vi "Controller Build FA Blocks and Send to Fast Archiver Data Loop.vi"(5 "Number of Blocks":u32, 7 "FA Data (Zeroed)":sgl[][](array[numeric]), 8 "Timestamp":u64, 9 "FC Marker":u32, 10 "FA Data (BPM Readings / PS Readings / PS Setpoints)":dbl[](array[numeric]), 11 "Queue in":refnum<queue>) -> ()   [LabVIEW 2011, in "Controller VIs.lvlib"]
uses:
  Controller VIs.lvlib
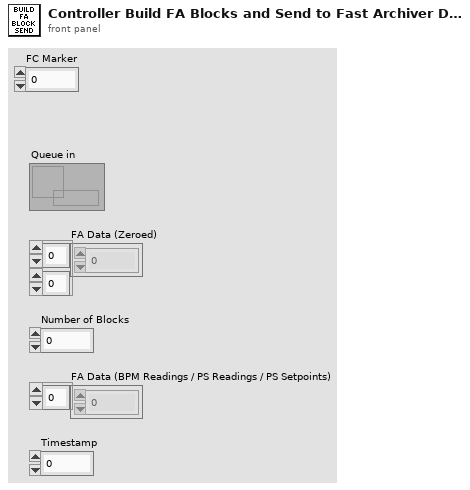
[diagram p1: front panel]
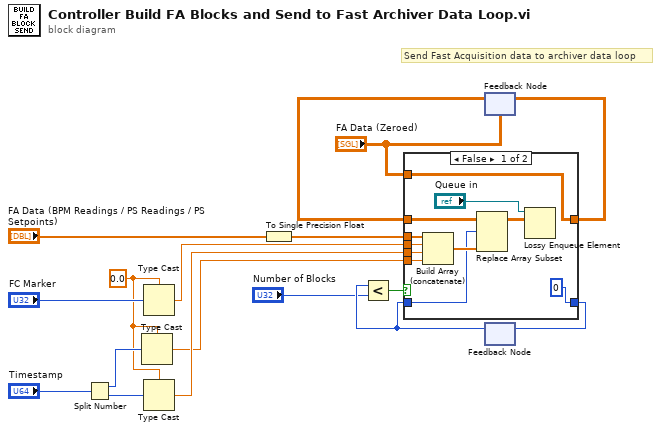
[diagram p0: block diagram]
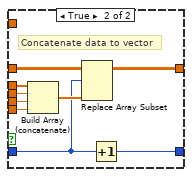
[diagram p2: hidden frame]
diagram:
  w2 = sgl 0.0 ("single precision float")
  # "Send Fast Acquisition data to archiver data loop"
  n1 = Split Number(x="Timestamp") -> (hi(x)=w15:u32, lo(x)=w14:u32)
  n2 = Type Cast(type=w2, x=w15) -> (*(type *) &x=w16:sgl)
  n3 = Type Cast(type=w2, x="FC Marker") -> (*(type *) &x=w1:sgl)
  n4 = Type Cast(type=w2, x=w14) -> (*(type *) &x=w17:sgl)
  n5 = To Single Precision Float(number="FA Data (BPM Readings / PS Readings / PS Setpoints)") -> (single precision float=w13:sgl[])
  n6 = feedback #1("FA Data (Zeroed)") -> (w7:sgl[][])
  n7 = feedback #2() -> (w11:i32)  [unwired: 1 in]
  n8 = Less?(x=w11, y="Number of Blocks") -> (x < y?=w9:bool)
  n9 = case shown="False" w9 {
    tunnel: [0 ("x+1") w35] -> w8
    tunnel: [w21 w34] -> w6
    tunnel: w7 -> [w28 w37]
    tunnel: w11 -> [w25 w33]
    tunnel: w17 -> [w19 w30]
    tunnel: w13 -> [w23 w32]
    tunnel: w16 -> [w20 w31]
    tunnel: "FA Data (Zeroed)" -> [w21 _]
    tunnel: w1 -> [w18 w29]
    frame False {
      n10 = Build Array (concatenate)(w23, w18, w19, w20) -> (w27:sgl[])
      n11 = Replace Array Subset(array=w28, new element=w27, index (row)=w25) -> (w24:sgl[][])  [unwired: 1 in]
      n12 = Lossy Enqueue Element(queue="Queue in", element=w24) -> ()  [unwired: 1 in, 4 out]
    }
    frame True {
      # "Concatenate data to vector"
      n13 = Build Array (concatenate)(w32, w29, w30, w31) -> (w36:sgl[])
      n14 = Replace Array Subset(array=w37, new element=w36, index (row)=w33) -> (w34:sgl[][])  [unwired: 1 in]
      n15 = Increment(x=w33) -> (x+1=w35:i32)
    }
  }
  n16 = feedback-in #1(w6) -> ()
  n17 = feedback-in #2(w8) -> ()
